vi "Meas Create Data Folder.vi"(8 "error in":errorcluster, 11 "sequence item":T1) -> (0 "error out":errorcluster)   [LabVIEW 2013]
doc: "Takes file path (either full or with file name base), extracts folder path, checks if it exists and creates new one in not exist yet."
uses:
  Meas Sequence Item.ctl
  Meas Sampling Configuration.ctl
  adc/ADC Trig Config.ctl
  adc/ADC Trig Mode Source.ctl
  adc/ADC Trig Coupling.ctl
  adc/ADC Trig Slope.ctl
  processing/QWTB/Meas Proc QWTB Algorithm Parameter Data.ctl
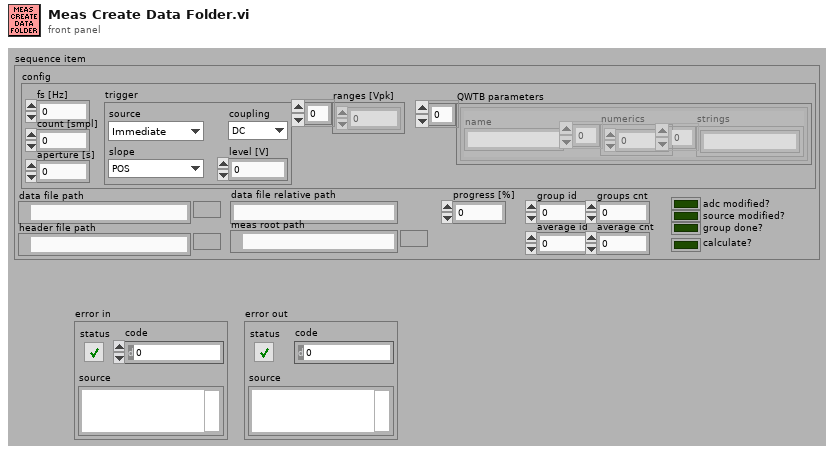
[diagram p1: front panel]
types:
  T1 = typedef "Meas Sequence Item.ctl" = cluster{"config":T2, "data file path":path, "header file path":path, "group id":i32, "average id":i32, "group done?":bool, "adc modified?":bool, "source modified?":bool, "progress [%]":dbl, "groups cnt":i32, "average cnt":i32, "data file relative path":string, "meas root path":path, "calculate?":bool}
  T2 = typedef "Meas Sampling Configuration.ctl" = cluster{"fs [Hz]":dbl, "count [smpl]":i64, "aperture [s]":dbl, "trigger":T3, "ranges [Vpk]":dbl[], "QWTB parameters":T7[]}
  T3 = typedef "ADC Trig Config.ctl" = cluster{"source":T4, "level [V]":dbl, "coupling":T5, "slope":T6}
  T4 = typedef "ADC Trig Mode Source.ctl" = enum16{"Immediate", "External", "Level"}
  T5 = typedef "ADC Trig Coupling.ctl" = enum16{"DC", "AC"}
  T6 = typedef "ADC Trig Slope.ctl" = enum16{"POS", "NEG"}
  T7 = typedef "Meas Proc QWTB Algorithm Parameter Data.ctl" = cluster{"name":string, "numerics":dbl[], "strings":string[]}
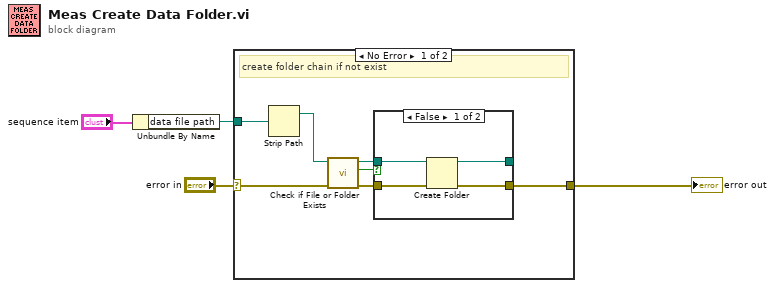
[diagram p0: block diagram]
diagram:
  n1 = Unbundle By Name("sequence item") -> ("data file path"=w1:path)
  n2 = case shown="No Error" "error in" {
    selector: "error in" -> [w10 w18]
    tunnel: w1 -> [w11 _]
    tunnel: [w5 w18] -> w4
    frame No Error {
      # "create folder chain if not exist"
      n3 = Strip Path(path=w11) -> (stripped path=w9:path)  [unwired: 1 out]
      n4 = call <vilib>:"Check if File or Folder Exists.vi"("error in (no error)"=w10, "path"=w9) -> ("error out"=w8:errorcluster, "file or folder exists?"=w6:bool, "dup path"=w7:path)  [unwired: 7 in]
      n5 = case shown="False" w6 {
        tunnel: w8 -> [w15 w16]
        tunnel: w7 -> [w14 w17]
        tunnel: [w13 w16] -> w5
        tunnel: [w12 w17] -> _
        frame False {
          n6 = Create Folder(path (use dialog)=w14, error in=w15) -> (created path=w12:path, error out=w13:errorcluster)  [unwired: 1 in, 1 out]
        }
        frame True {
        }
      }
    }
    frame Error {
    }
  }
  "error out" <- w4
